vi "get_visitor.vi"(0 "HGF_FGV_Visitor":refnum<class "HGF_FGV_Visitor.lvclass">, 5 "error in (no error)":errorcluster) -> (14 "dup HGF_FGV_Visitor":refnum<class "HGF_FGV_Visitor.lvclass">, 16 "visitor":refnum<class "HGF_Visitor.lvclass">, 19 "error out":errorcluster)   [LabVIEW 2012, in "HGF_FGV.lvlib" / "HGF_FGV_Visitor.lvclass"]
uses:
  HGF_FGV_Visitor.lvclass
  HGF_Visitor/HGF_Visitor.lvclass
  HGF_FGV_Visitor.lvclass/HGF_FGV_Visitor.ctl
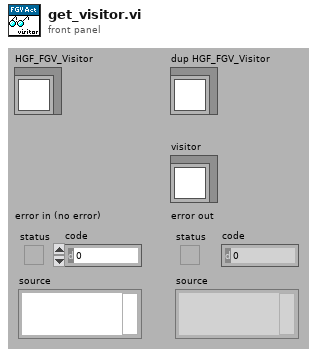
[diagram p1: front panel]
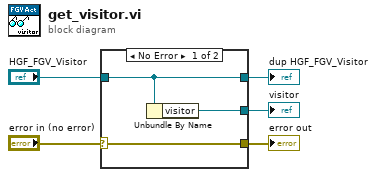
[diagram p0: block diagram]
diagram:
  n1 = case shown="No Error" "error in (no error)" {
    selector: "error in (no error)" -> [w8 w9]
    tunnel: [w8 w9] -> w4
    tunnel: [w7 w10] -> w2
    tunnel: "HGF_FGV_Visitor" -> [w7 w10]
    tunnel: [w6 _] -> w1
    frame No Error {
      n2 = Unbundle By Name(w7) -> ("visitor"=w6:refnum<class "HGF_Visitor.lvclass">)
    }
    frame Error {
    }
  }
  "error out" <- w4
  "dup HGF_FGV_Visitor" <- w2
  "visitor" <- w1
